vi "Graphics-Distance to Line Segment.vi"(0 "segmentStart":cluster{"x":i16, "y":i16}, 5 "segmentEnd":cluster{"x":i16, "y":i16}, 9 "point":cluster{"x":i16, "y":i16}) -> (8 "distance":dbl)   [LabVIEW 2020]
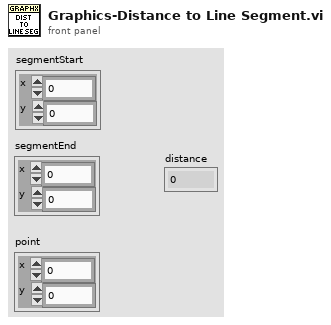
[diagram p1: front panel]
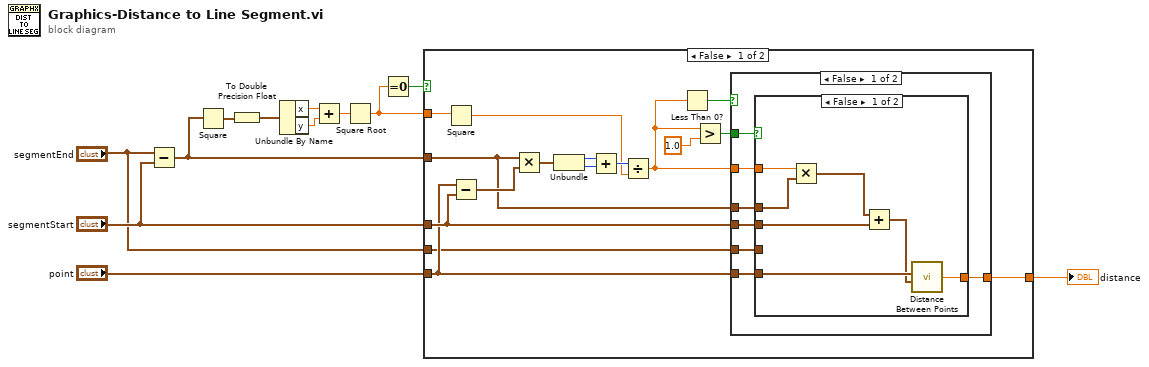
[diagram p0: block diagram]
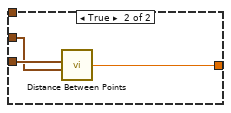
[diagram p2: hidden frame]
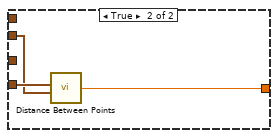
[diagram p3: hidden frame]
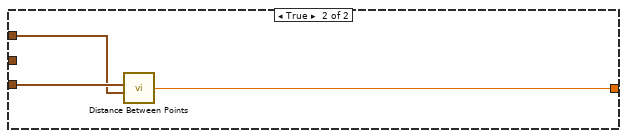
[diagram p4: hidden frame]
diagram:
  n1 = Subtract(x="segmentEnd", y="segmentStart") -> (x-y=w4:cluster{"x":i16, "y":i16})
  n2 = Square(x=w4) -> (x^2=w9:cluster{"x":i16, "y":i16})
  n3 = To Double Precision Float(number=w9) -> (double precision float=w1:cluster{"x":dbl, "y":dbl})
  n4 = Unbundle By Name(w1) -> ("x"=w10:dbl, "y"=w11:dbl)
  n5 = Add(x=w10, y=w11) -> (x+y=w12:dbl)
  n6 = Square Root(x=w12) -> (sqrt(x)=w3:dbl)
  n7 = Equal To 0?(x=w3) -> (x = 0?=w8:bool)
  n8 = case shown="False" w8 {
    tunnel: "point" -> [w19 w51]
    tunnel: "segmentStart" -> [w20 w50]
    tunnel: [w18 w49] -> w5
    tunnel: w4 -> [w13 _]
    tunnel: w3 -> [w23 _]
    tunnel: "segmentEnd" -> [w15 _]
    frame False {
      n9 = Square(x=w23) -> (x^2=w22:dbl)
      n10 = Subtract(x=w19, y=w20) -> (x-y=w28:cluster{"x":i16, "y":i16})
      n11 = Multiply(x=w13, y=w28) -> (x*y=w27:cluster{"x":i16, "y":i16})
      n12 = Unbundle(w27) -> ("x"=w26:i16, "y"=w25:i16)
      n13 = Add(x=w26, y=w25) -> (x+y=w24:i16)
      n14 = Divide(x=w24, y=w22) -> (x/y=w14:dbl)
      n15 = Less Than 0?(x=w14) -> (x < 0?=w21:bool)
      n16 = Greater?(x=w14, y=1.0) -> (0:w16:bool)
      n17 = case shown="False" w21 {
        tunnel: w20 -> [w30 w47]
        tunnel: w19 -> [w34 w48]
        tunnel: [w32 w46] -> w18
        tunnel: w16 -> [w35 _]
        tunnel: w15 -> [w33 _]
        tunnel: w14 -> [w31 _]
        tunnel: w13 -> [w29 _]
        frame False {
          n18 = case shown="False" w35 {
            tunnel: w34 -> [w42 w45]
            tunnel: w33 -> [_ w44]
            tunnel: [w41 w43] -> w32
            tunnel: w31 -> [w38 _]
            tunnel: w30 -> [w40 _]
            tunnel: w29 -> [w37 _]
            frame False {
              n19 = Multiply(x=w38, y=w37) -> (x*y=w36:cluster{"x":dbl, "y":dbl})
              n20 = Add(x=w36, y=w40) -> (x+y=w39:cluster{"x":dbl, "y":dbl})
              n21 = call "Distance Between Points.vi"("B"=w39, "A"=w42) -> ("distance"=w41:dbl)  [unwired: 4 in]
            }
            frame True {
              n22 = call "Distance Between Points.vi"("B"=w44, "A"=w45) -> ("distance"=w43:dbl)  [unwired: 4 in]
            }
          }
        }
        frame True {
          n23 = call "Distance Between Points.vi"("B"=w47, "A"=w48) -> ("distance"=w46:dbl)  [unwired: 4 in]
        }
      }
    }
    frame True {
      n24 = call "Distance Between Points.vi"("B"=w50, "A"=w51) -> ("distance"=w49:dbl)  [unwired: 4 in]
    }
  }
  "distance" <- w5
